vi "Set Energize Enable.vi"(0 "object in":refnum<class "HPS-17000-PowerModule.lvclass">, 5 "energize":bool, 11 "Error In":errorcluster) -> (4 "object out":refnum<class "HPS-17000-PowerModule.lvclass">, 15 "Error Out":errorcluster)   [LabVIEW 2023, in "HPS-17000-PowerModule.lvlib" / "HPS-17000-PowerModule.lvclass"]
uses:
  HPS-17000-PowerModule.lvclass
  <instrlib>/HPS-17000/Internal/Set Energized Multi.vi
  <instrlib>/HPS-17000/HPS-17000.lvclass
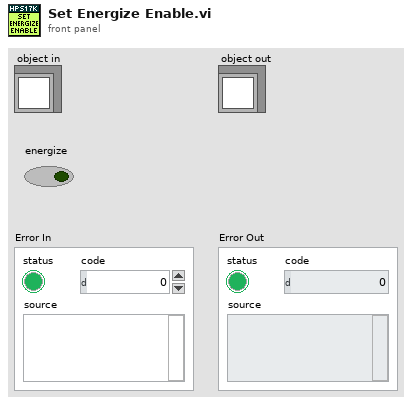
[diagram p1: front panel]
types:
  T1 = typedef "HPS-17000-PowerModule.lvlib/HPS-17000-PowerModule.lvclass/ObjectAttributes.ctl" = cluster{"HPS17000 IP Addresses":string[], "HPS Topology":enum16{"SINGLE", "MULTI"}, "GM ID":string, "TSN NIC IP Address":string, "HPS17000 Refs":refnum<class "HPS-17000.lvclass">[], "Stream Queues":refnum<queue>[], "connected":bool, "reserved":bool, "events":T2, "nibatterycycler_grpc_Setpoint":T3, "last timestamp":i64, "setpoint stream config":T4, "mode":T5, "range":T6}
  T2 = typedef "HPS-17000.lvclass/Multi-Cycler Events.ctl" = cluster{"heartbeats events":refnum<user-event>[], "faults events":refnum<user-event>[], "network sync event":refnum<user-event>[], "setpoint status event":refnum<user-event>[]}
  T3 = typedef "NI_BC_client.lvlib/nibatterycycler_grpc_Setpoint.ctl" = cluster{"voltage":sgl, "current":sgl, "min_power":sgl, "max_power":sgl, "resistance":sgl}
  T4 = typedef "Cycler.lvclass/Setpoint Stream Basic Config.ctl" = cluster{"local address":string, "receiver port":u16}
  T5 = typedef "HPS-17000-PowerModule.lvlib/HPS-17000-PowerModule.lvclass/Mode.ctl" = u16
  T6 = typedef "PowerModuleInterface.lvlibp/PowerModuleInterface.lvclass/Range.ctl" = cluster{"Current Max (A)":dbl, "Current Min (A)":dbl, "Voltage Max (V)":dbl, "Voltage Min (V)":dbl}
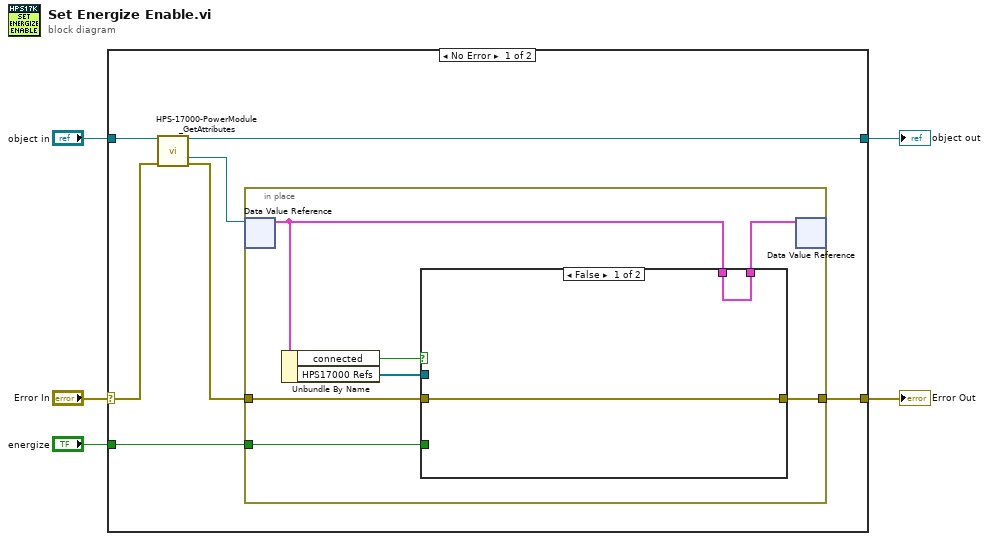
[diagram p0: block diagram]
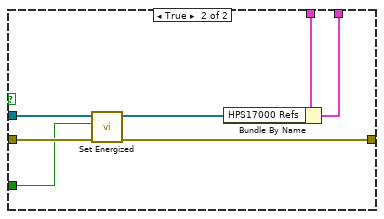
[diagram p2: hidden frame]
diagram:
  n1 = case shown="No Error" "Error In" {
    selector: "Error In" -> [w12 w30]
    tunnel: [w8 w29] -> w5
    tunnel: [w9 w30] -> w1
    tunnel: "object in" -> [w7 w29]
    tunnel: "energize" -> [w6 _]
    frame No Error {
      n2 = call "HPS-17000-PowerModule_GetAttributes.vi"("reference in"=w7, "Error In"=w12) -> ("reference out"=w8:refnum<class "HPS-17000-PowerModule.lvclass">, "DataRef"=w11:refnum<data-value>, "Error Out"=w10:errorcluster)  [unwired: 10 in, 1 out]
      n3 = in-place {
        in-place-border: w10 -> [w17]
        in-place-border: [w16] -> w9
        in-place-border: w6 -> [w13]
        n4 = in-place-dvr #1(w11) -> (w18:T1)  [unwired: 1 out]
        n5 = Unbundle By Name(w18) -> ("connected"=w14:bool, "HPS17000 Refs"=w15:refnum<class "HPS-17000.lvclass">[])
        n6 = case shown="False" w14 {
          tunnel: [w21 w28] -> w19
          tunnel: w18 -> [w21 w27]
          tunnel: w17 -> [w20 w24]
          tunnel: [w20 w23] -> w16
          tunnel: w15 -> [_ w26]
          tunnel: w13 -> [_ w22]
          frame False {
          }
          frame True {
            n7 = call-poly <instrlib>:"Set Energized.vi"("error in"=w24, "energize (T)"=w22, "cycler refs in"=w26) -> ("error out"=w23:errorcluster, "cycler refs out"=w25:refnum<class "HPS-17000.lvclass">[])  [unwired: 7 in]
            n8 = Bundle By Name(cluster=w27, "HPS17000 Refs"=w25) -> (w28:T1)
          }
        }
        n9 = in-place-dvr #1(w19) -> ()  [unwired: 2 out]
      }
    }
    frame Error {
    }
  }
  "Error Out" <- w1
  "object out" <- w5
